vi "Convert  Sample to second.vi"(8 "Sample rate":i32=1, 10 "samples collected":i32) -> (0 "Second":u8, 1 "Duration":string, 2 "Minute":u8, 3 "Hour":u8)   [LabVIEW 2017]
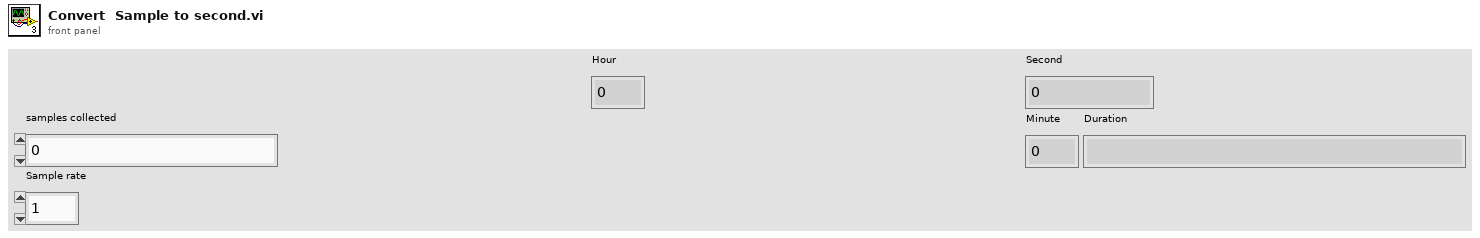
[diagram p1: front panel]
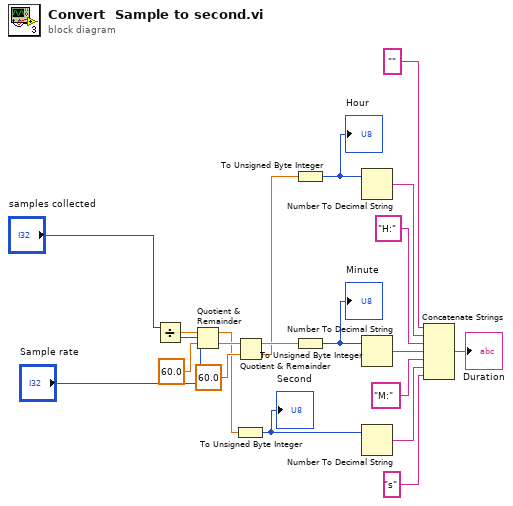
[diagram p0: block diagram]
diagram:
  n1 = Divide(x="samples collected", y="Sample rate") -> (x/y=w19:dbl)
  n2 = Quotient & Remainder(x=w19, y=60.0) -> (x-y*floor(x/y)=w15:dbl, floor(x/y)=w17:dbl)
  n3 = To Unsigned Byte Integer(number=w15) -> (unsigned 8bit integer=w12:u8)
  "Second" <- w12
  n4 = Quotient & Remainder(x=w17, y=60.0) -> (x-y*floor(x/y)=w14:dbl, floor(x/y)=w13:dbl)
  n5 = To Unsigned Byte Integer(number=w13) -> (unsigned 8bit integer=w11:u8)
  "Hour" <- w11
  n6 = To Unsigned Byte Integer(number=w14) -> (unsigned 8bit integer=w10:u8)
  "Minute" <- w10
  n7 = Number To Decimal String(number=w11) -> (decimal integer string=w8:string)  [unwired: 1 in]
  n8 = Number To Decimal String(number=w10) -> (decimal integer string=w7:string)  [unwired: 1 in]
  n9 = Number To Decimal String(number=w12) -> (decimal integer string=w6:string)  [unwired: 1 in]
  n10 = Concatenate Strings("" ("string"), w8, "H:" ("string"), w7, "M:" ("string"), w6, "s" ("string")) -> (→"Duration":string)
